vi "Setup.vi"(8 "error in (no error)":errorcluster, 11 "Rig Test In":refnum<class "Application Test.lvclass">) -> (0 "error out":errorcluster, 3 "Rig Test Out":refnum<class "Application Test.lvclass">)   [LabVIEW 2020, in "Application Test.lvclass"]
uses:
  Application Test.lvclass
  C:/Git/astemes-triarc-framework/source/Framework Test/Base Class Test/Base Test.lvclass
  Framework/Application/Application.lvclass
  C:/Git/astemes-triarc-framework/source/Framework/Base/Base.lvclass
  Base Class Test/Base Test.lvclass/Base Test.ctl
  Application Test.lvclass/Application Test.ctl
  Base Class Test/Base Test.lvclass
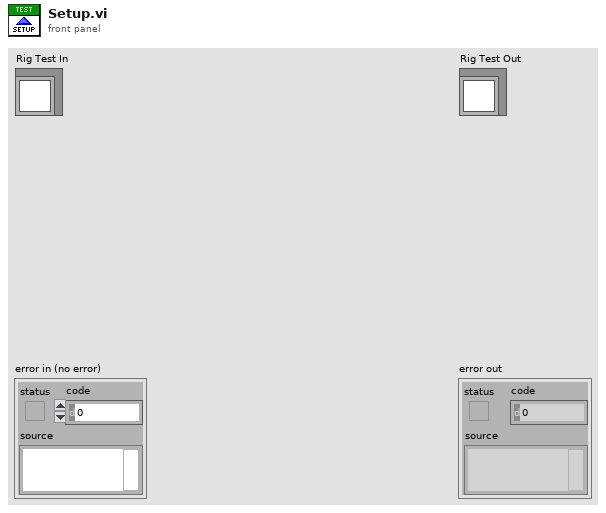
[diagram p1: front panel]
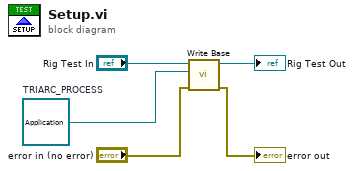
[diagram p0: block diagram]
diagram:
  w3 = refnum<class "Application.lvclass"> refnum  # TRIARC_PROCESS
  n1 = call "Write Base.vi"("error in (no error)"="error in (no error)", "Base"=w3, "Base Class Test In"="Rig Test In") -> ("error out"=→"error out":errorcluster, "Base Class Test Out"=→"Rig Test Out":refnum<class "Application Test.lvclass">)  [unwired: 7 in]
